vi "Get Button Type.vi"(8 "error in (no error)":errorcluster, 11 "Button in":refnum<class "Button.lvclass">) -> (0 "error out":errorcluster, 2 "Type":T1, 3 "Button out":refnum<class "Button.lvclass">)   [LabVIEW 2012, in "Button.lvclass"]
uses:
  Button.lvclass
  Type Defs/Button Type.ctl
  Button.lvclass/Button.ctl
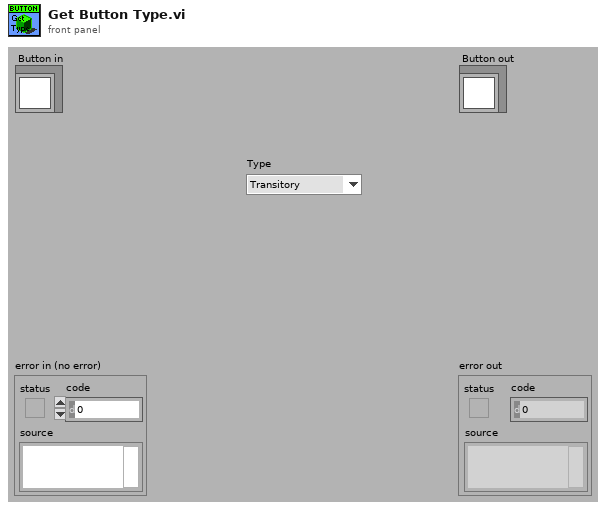
[diagram p1: front panel]
types:
  T1 = typedef "Button.lvclass/Button Type.ctl" = enum16{"Transitory", "Latching"}
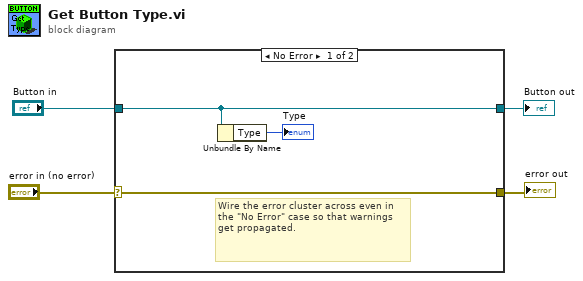
[diagram p0: block diagram]
diagram:
  n1 = case shown="No Error" "error in (no error)" {
    selector: "error in (no error)" -> [w7 w9]
    tunnel: [w7 w9] -> w3
    tunnel: [w6 w8] -> w1
    tunnel: "Button in" -> [w6 w8]
    frame No Error {
      # "Wire the error cluster across even in the \"No Error\" case so that warnings get propagated."
      n2 = Unbundle By Name(w6) -> ("Type"=→"Type":T1)
    }
    frame Error {
    }
  }
  "error out" <- w3
  "Button out" <- w1
